vi "Binary to decimal.vi"() -> ()   [LabVIEW 2015]
panel:
  out "x":i32
  out "number":i64
  out "Array":bool[](array[boolean])
  out "size(s)":i32
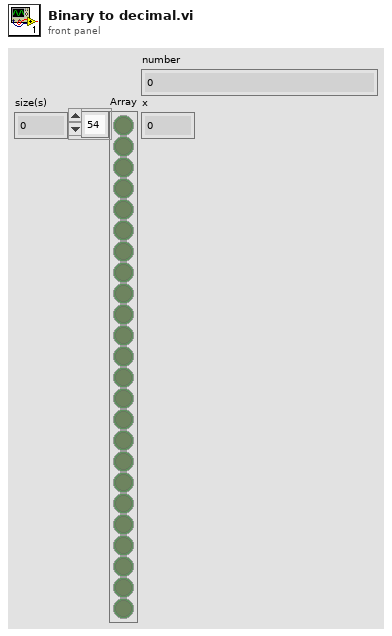
[diagram p1: front panel]
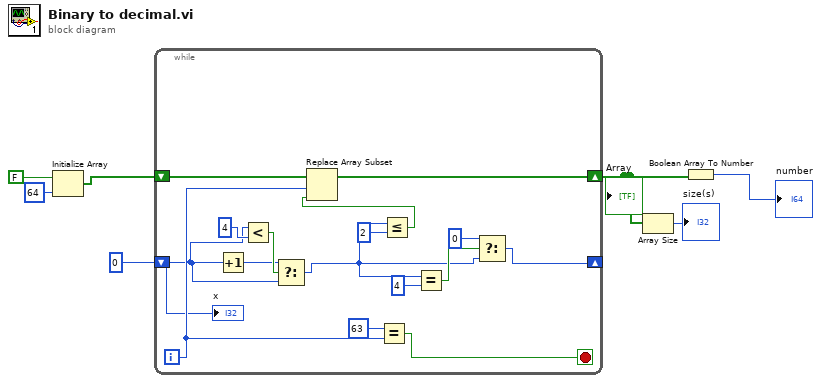
[diagram p0: block diagram]
diagram:
  n1 = Initialize Array(FALSE, 64 ("dimension size")) -> (w5:bool[])
  n2 = while {
    shift-right: [w22] -> w3
    shift-left: w5 -> [w23]
    shift-right: [w9] -> _
    shift-left: 0 ("x") -> [w14]
    i -> [w21]
    stop <- w19 stop-if-true
    n3 = Increment(x=w14) -> (x+1=w15:i32)
    n4 = Less?(x=w14, y=4 ("x")) -> (x < y?=w18:bool)
    n5 = Select(t=w15, s=w18, f=w14) -> (s? t:f=w11:i32)
    n6 = Equal?(x=63, y=w21) -> (x = y?=w19:bool)
    n7 = Less Or Equal?(x=w11, y=2) -> (x <= y?=w8:bool)
    n8 = Replace Array Subset(array=w23, new element=w8, index=w21) -> (w22:bool[])
    n9 = Equal?(x=w11, y=4) -> (x = y?=w12:bool)
    n10 = Select(t=0, s=w12, f=w11) -> (s? t:f=w9:i32)
    "x" <- w14
  }
  "Array" <- w3
  n11 = Array Size(array=w3) -> (size(s)=→"size(s)":i32)
  n12 = Boolean Array To Number(Boolean array=w3) -> (number=→"number":i64)
